vi "RightClickUpdate Delta.vi"(8 "error in (no error)":errorcluster, 10 "Refs":T13, 11 "Loop data in":T2={"TitleCollapse"=refnum, "MouseDownState"=enum."Idle", "RightClickCache"={"Mod"={"Ctrl"=FALSE, "Shift"=FALSE}, "CoordsStart"={"Horizontal"=0, "Vertical"=0}, "CoordsEnd"={"Horizontal"=0, "Vertical"=0}, "PlotAreaBounds"={"Left"=10, "Top"=10, "Right"=0, "Bottom"=0}, "slice"=[]}, "ZoomCache"={"SuppressedPlots"=[], "LeftAxis"={"NeedsRevert?"=FALSE, "Scale Fit"=0, "Range"={"Minimum"=0.0, "Maximum"=0.0, "Increment"=0.0, "Minor Increment"=0.0, "Start"=0.0}}, "RightAxis"={"NeedsRevert?"=FALSE, "Scale Fit"=0, "Range"={"Minimum"=0.0, "Maximum"=0.0, "Increment"=0.0, "Minor Increment"=0.0, "Start"=0.0}}, "Mod"={"Shift"=FALSE}}, "UpdateTime"=0.0, "keyboard"=refnum, "visible?"=FALSE}) -> (0 "error out":errorcluster, 2 "cells":T1[][](array[typedef]), 3 "Loop data out":T2={"TitleCollapse"=refnum, "MouseDownState"=enum."Idle", "RightClickCache"={"Mod"={"Ctrl"=FALSE, "Shift"=FALSE}, "CoordsStart"={"Horizontal"=0, "Vertical"=0}, "CoordsEnd"={"Horizontal"=0, "Vertical"=0}, "PlotAreaBounds"={"Left"=10, "Top"=10, "Right"=0, "Bottom"=0}, "slice"=[]}, "ZoomCache"={"SuppressedPlots"=[], "LeftAxis"={"NeedsRevert?"=FALSE, "Scale Fit"=0, "Range"={"Minimum"=0.0, "Maximum"=0.0, "Increment"=0.0, "Minor Increment"=0.0, "Start"=0.0}}, "RightAxis"={"NeedsRevert?"=FALSE, "Scale Fit"=0, "Range"={"Minimum"=0.0, "Maximum"=0.0, "Increment"=0.0, "Minor Increment"=0.0, "Start"=0.0}}, "Mod"={"Shift"=FALSE}}, "UpdateTime"=0.0, "keyboard"=refnum, "visible?"=FALSE}, 4 "Row Headers":string[](array[string]), 6 "Column Headers":string[](array[string]))   [LabVIEW 2021, in "RocketPlot.lvlib"]
uses:
  RocketPlot.lvlib
  TypeDefs/Plot UI references.ctl
  Classes/RocketPlotHandle/RocketPlotHandle.lvclass
  <userlib>/bjustice/TipStripOOPanel/Classes/TipPanelHandle/TipPanelHandle.lvclass
  TypeDefs/Plot top row.ctl
  TypeDefs/plot while loop data.ctl
  CollapsePanel/CollapsePanel.lvclass
  TypeDefs/MouseDownState.ctl
  TypeDefs/RightClickCache.ctl
  TypeDefs/RightClickCache PlatMod.ctl
  <vilib>/Utility/miscctls.llb/LVPoint32TypeDef.ctl
  <vilib>/Utility/miscctls.llb/LVRectTypeDef.ctl
  TypeDefs/Slice average.ctl
  TypeDefs/ZoomCache.ctl
  TypeDefs/RangeCache.ctl
  <vilib>/Utility/miscctls.llb/LVRangeTypeDef.ctl
  TypeDefs/ZoomCache PlatMod.ctl
  Classes/TipTablePanel/cell cache.ctl
  Plot scale refnum to LUT name.vi
  Classes/TipTablePanel/TipTablePanel.lvclass
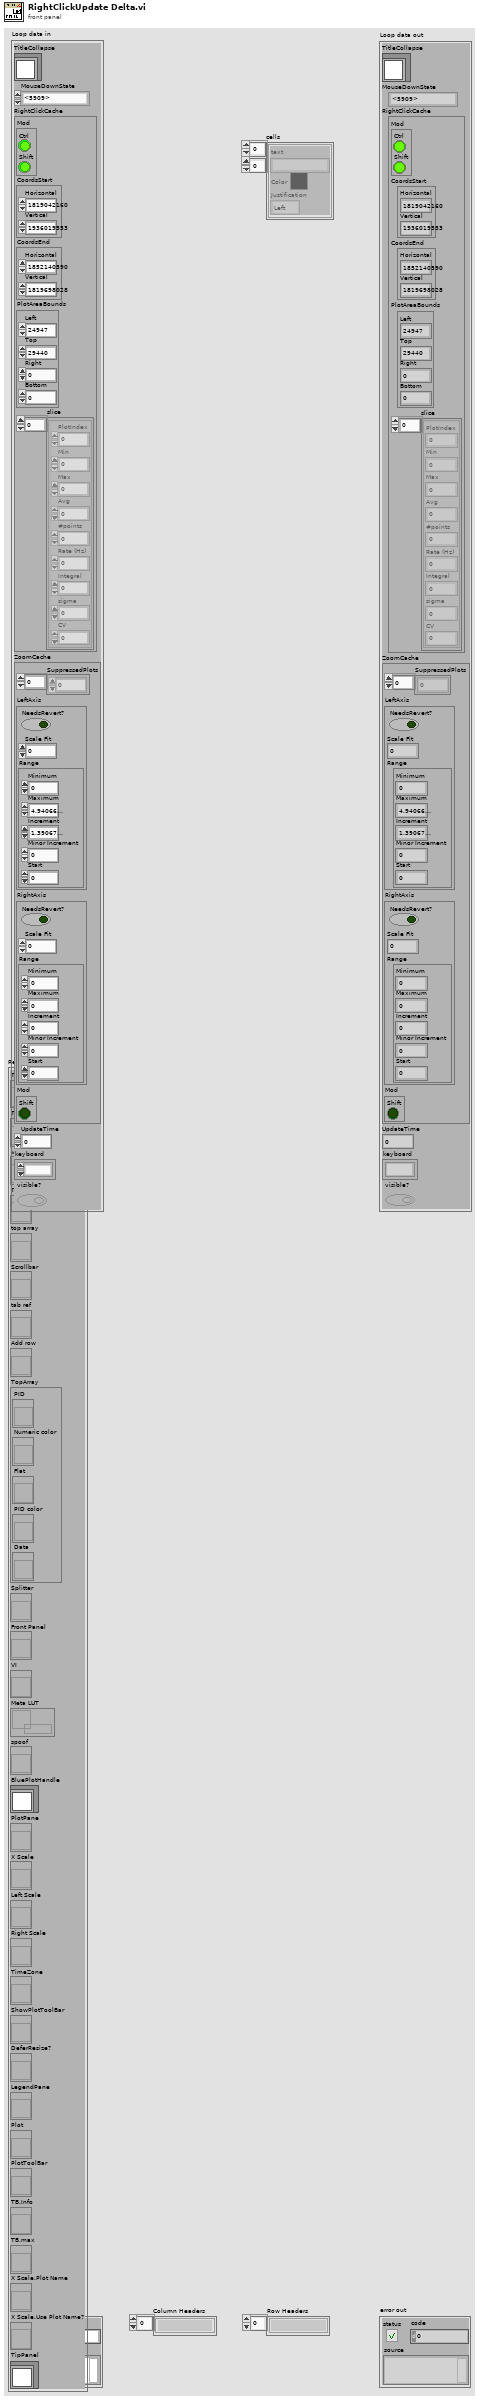
[diagram p1: front panel]
types:
  T1 = typedef "RocketPlot.lvlib/TipTablePanel.lvclass/cell cache.ctl" = cluster{"text":string, "Color":u32, "Justification":enum16{"Left", "Center", "Right"}}
  T2 = typedef "RocketPlot.lvlib/plot while loop data.ctl" = cluster{"TitleCollapse":refnum<class "CollapsePanel.lvclass">, "MouseDownState":T3, "RightClickCache":T4, "ZoomCache":T9, "UpdateTime":dbl, "keyboard":refnum<k1>, "visible?":bool}
  T3 = typedef "RocketPlot.lvlib/MouseDownState.ctl" = enum16{"Idle", "Pan", "Zoom", "Zoom-Post", "RightClick"}
  T4 = typedef "RocketPlot.lvlib/RightClickCache.ctl" = cluster{"Mod":T5, "CoordsStart":T6, "CoordsEnd":T6, "PlotAreaBounds":T7, "slice":T8[]}
  T5 = typedef "RocketPlot.lvlib/RightClickCache PlatMod.ctl" = cluster{"Ctrl":bool, "Shift":bool}
  T6 = typedef "LVPoint32TypeDef.ctl" = cluster{"Horizontal":i32, "Vertical":i32}
  T7 = typedef "LVRectTypeDef.ctl" = cluster{"Left":i16, "Top":i16, "Right":i16, "Bottom":i16}
  T8 = typedef "RocketPlot.lvlib/Slice average.ctl" = cluster{"PlotIndex":i32, "Min":dbl, "Max":dbl, "Avg":dbl, "#points":u32, "Rate (Hz)":dbl, "Integral":dbl, "sigma":dbl, "CV":dbl}
  T9 = typedef "RocketPlot.lvlib/ZoomCache.ctl" = cluster{"SuppressedPlots":i32[], "LeftAxis":T10, "RightAxis":T10, "Mod":T12}
  T10 = typedef "RocketPlot.lvlib/RangeCache.ctl" = cluster{"NeedsRevert?":bool, "Scale Fit":u8, "Range":T11}
  T11 = typedef "LVRangeTypeDef.ctl" = cluster{"Minimum":dbl, "Maximum":dbl, "Increment":dbl, "Minor Increment":dbl, "Start":dbl}
  T12 = typedef "RocketPlot.lvlib/ZoomCache PlatMod.ctl" = cluster{"Shift":bool}
  T13 = typedef "RocketPlot.lvlib/Plot UI references.ctl" = cluster{"Title":refnum<vi>, "Title?":refnum<vi>, "Visible sidebar?":refnum<vi>, "Time to Plot":refnum<vi>, "top array":refnum<vi>, "Scrollbar":refnum<vi>, "tab ref":refnum<vi>, "Add row":refnum<vi>, "TopArray":cluster{"PID":refnum<vi>, "Numeric color":refnum<vi>, "Flat":refnum<vi>, "PID color":refnum<vi>, "Data":refnum<vi>}, "Splitter":refnum<vi>, "Front Panel":refnum<vi>, "VI":refnum<vi>, "Meta LUT":refnum<data-value>, "spoof":refnum<vi>, "BluePlotHandle":refnum<class "RocketPlotHandle.lvclass">, "PlotPane":refnum<vi>, "X Scale":refnum<vi>, "Left Scale":refnum<vi>, "Right Scale":refnum<vi>, "TimeZone":refnum<vi>, "ShowPlotToolBar":refnum<vi>, "DeferResize?":refnum<vi>, "LegendPane":refnum<vi>, "Plot":refnum<vi>, "PlotToolBar":refnum<vi>, "TB.Info":refnum<vi>, "TB.max":refnum<vi>, "X Scale.Plot Name":refnum<vi>, "X Scale.Use Plot Name?":refnum<vi>, "TipPanel":refnum<class "TipPanelHandle.lvclass">}
  T14 = typedef "RocketPlot.lvlib/Plot scale meta JSON.ctl" = cluster{"Type":T15, "Grid Colors:Major Color":u32, "Grid Colors:Minor Color":u32, "Style":u8, "Tick Colors:Tick Color":u32, "Tick Colors:Minor Tick Color":u32, "Format String":string, "State":T16, "AxisFocus":refnum<vi>}
  T15 = typedef "RocketPlot.lvlib/Plot axis.ctl" = enum16{"x axis", "left axis", "right axis"}
  T16 = typedef "RocketPlot.lvlib/Plot scale meta state.ctl" = cluster{"Visible":bool, "Focus":bool, "Multi-Y":bool}
  T17 = typedef "TimeZone.ctl" = enum16{"UTC", "Local"}
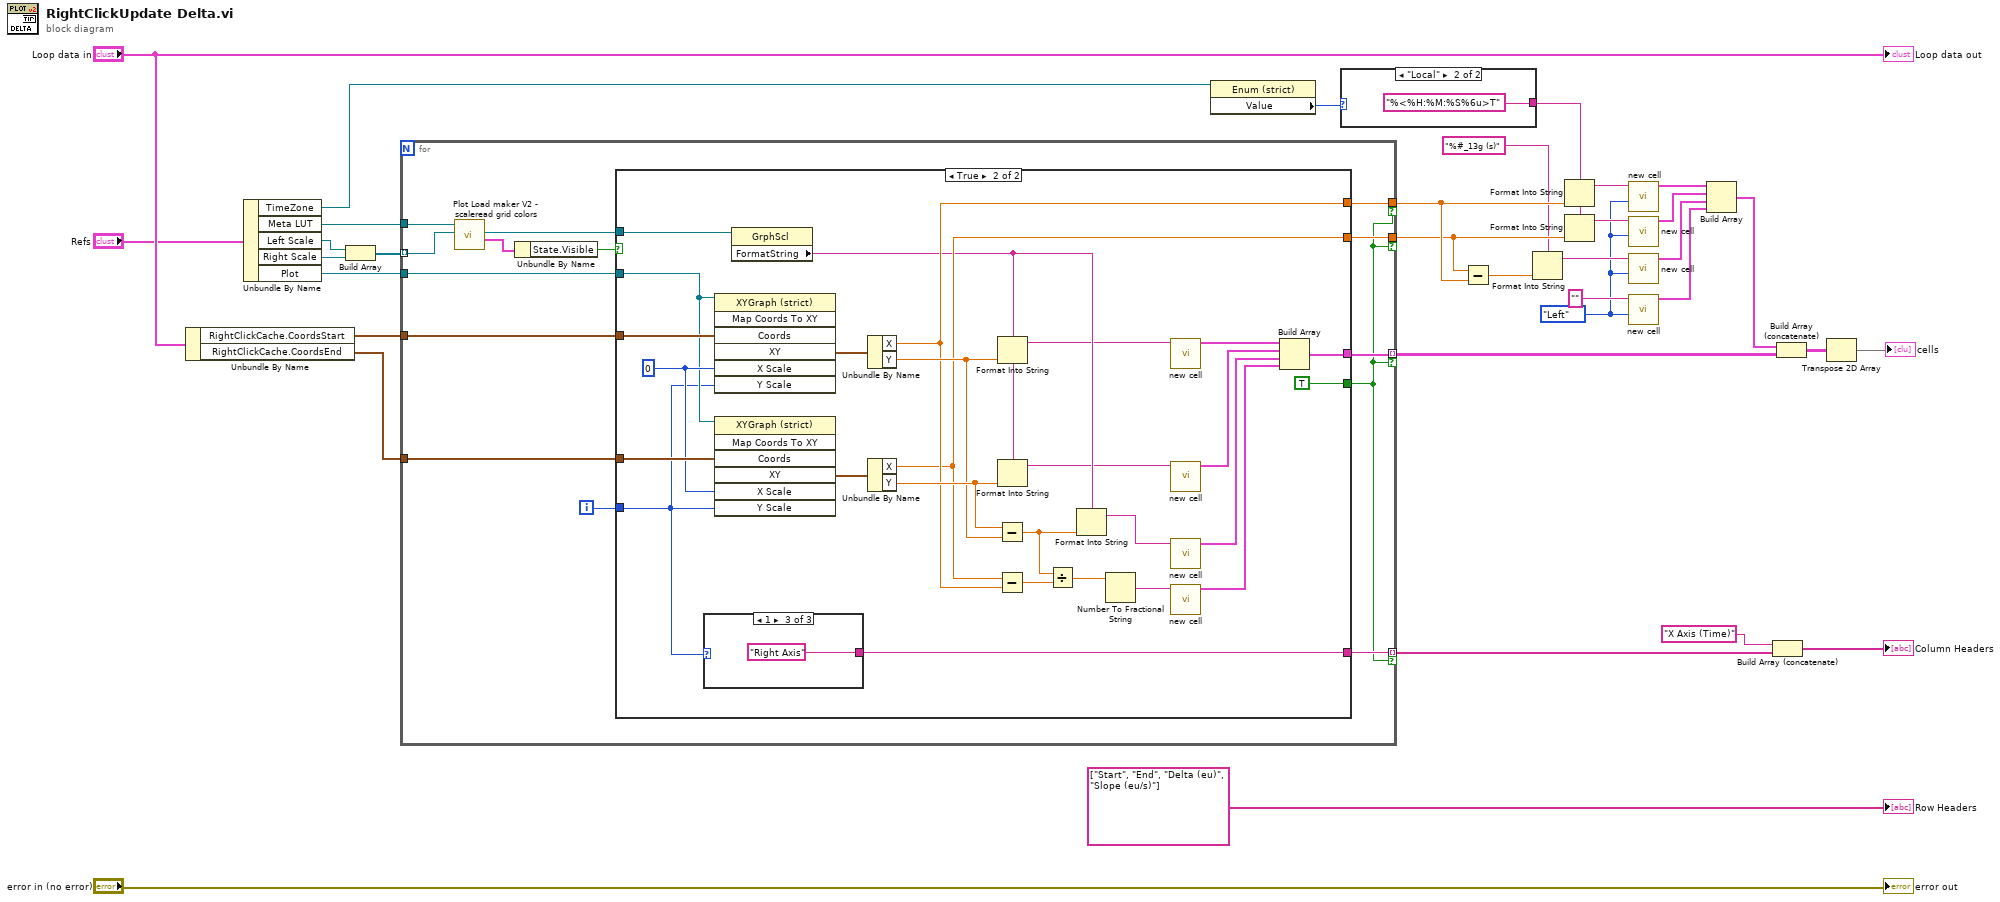
[diagram p0: block diagram]
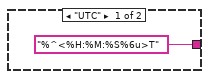
[diagram p2: hidden frame]
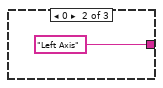
[diagram p5: hidden frame]
diagram:
  w6 = enum16{"Left", "Center", "Right"}."Left" ("Justification")
  n1 = Unbundle By Name("Loop data in") -> ("RightClickCache.CoordsStart"=w34:T6, "RightClickCache.CoordsEnd"=w33:T6)
  n2 = Unbundle By Name("Refs") -> ("TimeZone"=w14:refnum<vi>, "Meta LUT"=w26:refnum<data-value>, "Left Scale"=w29:refnum<vi>, "Right Scale"=w28:refnum<vi>, "Plot"=w25:refnum<vi>)
  n3 = Build Array(w29, w28) -> (w27:refnum<vi>[])
  n4 = for {
    tunnel: w34 -> [w48]
    tunnel: w33 -> [w47]
    tunnel: [w45] -> w23 mode=indexing if=w35
    tunnel: w27 -> [w43] mode=indexing
    tunnel: w26 -> [w44]
    tunnel: w25 -> [w40]
    tunnel: [w38] -> w20 mode=indexing if=w35
    tunnel: [w37] -> w16 if=w35
    tunnel: [w36] -> w15 if=w35
    i -> [w46]
    n5 = call "Plot Load maker V2 - scaleread grid colors.vi"("Scale reference"=w43, "Meta LUT"=w44) -> ("Scale LUT meta"=w42:T14, "Scale reference"=w39:refnum<vi>)  [unwired: 6 in, 2 out]
    n6 = Unbundle By Name(w42) -> ("State.Visible"=w41:bool)
    n7 = case shown="True" w41 {
      tunnel: w48 -> [_ w75]
      tunnel: w47 -> [_ w74]
      tunnel: w46 -> [_ w62]
      tunnel: [_ w66] -> w45
      tunnel: w40 -> [_ w65]
      tunnel: w39 -> [_ w64]
      tunnel: [_ TRUE] -> w35
      tunnel: [_ w61] -> w38
      tunnel: [_ w60] -> w37
      tunnel: [_ w59] -> w36
      frame False {
      }
      frame True {
        w73 = 0 ("X Scale")
        n8 = case shown="1" w62 {
          tunnel: [_ "Left Axis" ("String") "Right Axis" ("String")] -> w61
          frame Default {
          }
          frame 0 {
          }
          frame 1 {
          }
        }
        n9 = invoke class="XYGraph (strict)" method="Map Coords To XY"(reference=w65, "Coords"=w75, "X Scale"=w73, "Y Scale"=w62) -> ("XY"=w72:cluster{"X":dbl, "Y":dbl})  [unwired: 3 in, 6 out]
        n10 = invoke class="XYGraph (strict)" method="Map Coords To XY"(reference=w65, "Coords"=w74, "X Scale"=w73, "Y Scale"=w62) -> ("XY"=w71:cluster{"X":dbl, "Y":dbl})  [unwired: 3 in, 6 out]
        n11 = property class="GrphScl"(reference=w64) -> ("FormatString"=w57:string)  [unwired: 1 in, 2 out]
        n12 = Unbundle By Name(w72) -> ("X"=w60:dbl, "Y"=w69:dbl)
        n13 = Unbundle By Name(w71) -> ("X"=w59:dbl, "Y"=w70:dbl)
        n14 = Format Into String(format string=w57, w69) -> (resulting string=w56:string)  [unwired: 2 in, 1 out]
        n15 = Format Into String(format string=w57, w70) -> (resulting string=w54:string)  [unwired: 2 in, 1 out]
        n16 = Subtract(x=w70, y=w69) -> (x-y=w58:dbl)
        n17 = Subtract(x=w59, y=w60) -> (x-y=w68:dbl)
        n18 = Divide(x=w58, y=w68) -> (x/y=w67:dbl)
        n19 = Format Into String(format string=w57, w58) -> (resulting string=w52:string)  [unwired: 2 in, 1 out]
        n20 = Number To Fractional String(number=w67) -> (F-format string=w50:string)  [unwired: 3 in]
        n21 = call "new cell.vi"("String"=w56) -> ("cell"=w55:T1)  [unwired: 10 in]
        n22 = call "new cell.vi"("String"=w54) -> ("cell"=w53:T1)  [unwired: 10 in]
        n23 = call "new cell.vi"("String"=w52) -> ("cell"=w51:T1)  [unwired: 10 in]
        n24 = call "new cell.vi"("String"=w50) -> ("cell"=w49:T1)  [unwired: 10 in]
        n25 = Build Array(w55, w53, w51, w49) -> (w66:T1[])
      }
    }
  }
  n26 = property class="Enum (strict)"(reference=w14) -> ("Value"=w12:T17)  [unwired: 1 in, 2 out]
  n27 = case shown="\"Local\"" w12 {
    tunnel: ["%^<%H:%M:%S%6u>T" ("Format String") "%<%H:%M:%S%6u>T" ("Format String")] -> w11
    frame "UTC" {
    }
    frame "Local" {
    }
  }
  n28 = Subtract(x=w15, y=w16) -> (x-y=w17:dbl)
  n29 = Format Into String(format string="%#_13g (s)" ("Format String"), w17) -> (resulting string=w8:string)  [unwired: 2 in, 1 out]
  n30 = Format Into String(format string=w11, w16) -> (resulting string=w10:string)  [unwired: 2 in, 1 out]
  n31 = Format Into String(format string=w11, w15) -> (resulting string=w7:string)  [unwired: 2 in, 1 out]
  n32 = call "new cell.vi"("Justification"=w6, "String"=w10) -> ("cell"=w5:T1)  [unwired: 9 in]
  n33 = call "new cell.vi"("Justification"=w6, "String"=w7) -> ("cell"=w4:T1)  [unwired: 9 in]
  n34 = call "new cell.vi"("Justification"=w6, "String"=w8) -> ("cell"=w3:T1)  [unwired: 9 in]
  n35 = call "new cell.vi"("Justification"=w6, "String"="" ("format string")) -> ("cell"=w2:T1)  [unwired: 9 in]
  n36 = Build Array(w5, w4, w3, w2) -> (w22:T1[])
  n37 = Build Array (concatenate)("X Axis (Time)" ("String"), w20) -> (→"Column Headers":string[])
  n38 = Build Array (concatenate)(w22, w23) -> (w21:T1[][])
  n39 = Transpose 2D Array(2D array=w21) -> (transposed array=→"cells":T1[][])
  "error out" <- "error in (no error)"
  "Loop data out" <- "Loop data in"
  "Row Headers" <- string[] ["Start", "End", "Delta (eu)", "Slope (eu/s)"] ("Row Headers")
